vi "Get System Parameter by condition.vi"(8 "error in (no error)":errorcluster caption="错误输入（无错误）", 9 "Enable":bool[](array[boolean]), 10 "propertyName":string="BytesPersector", 11 "path":string="Win32_DiskDrive") -> (0 "error out":errorcluster caption="错误输出", 3 "Parameters":string[](array[string]))   [LabVIEW 2013, in "ManagementClass.lvclass"]
uses:
  ManagementClass.lvclass
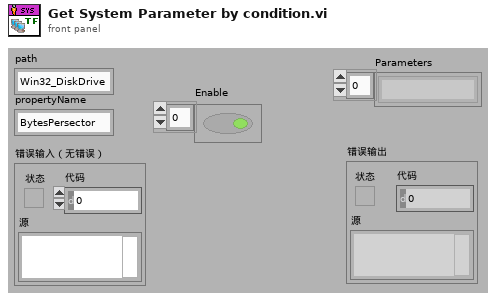
[diagram p1: front panel]
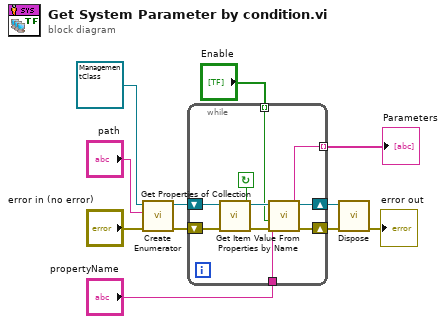
[diagram p0: block diagram]
diagram:
  n1 = call "Create Enumerator.vi"("error in (no error)"="error in (no error)", "path"="path", "ManagementClass 输入"=refnum<class "ManagementClass.lvclass"> refnum) -> ("error out"=w9:errorcluster, "ManagementClass 输出"=w10:refnum<class "ManagementClass.lvclass">)  [unwired: 7 in]
  n2 = while {
    shift-right: [w15] -> w7
    shift-left: w10 -> [w21]
    shift-right: [w16] -> w8
    shift-left: w9 -> [w18]
    tunnel: [w14] -> w2 mode=indexing
    tunnel: "propertyName" -> [w13]
    tunnel: "Enable" -> [w12] mode=indexing
    stop <- w20 continue-if-true
    n3 = call "Get Properties of Collection.vi"("error in (no error)"=w18, "ManagementClass 输入"=w21) -> ("error out"=w17:errorcluster, "非空"=w20:bool, "ManagementClass 输出"=w19:refnum<class "ManagementClass.lvclass">)  [unwired: 7 in]
    n4 = call "Get Item Value From Properties by Name.vi"("error in (no error)"=w17, "Enable"=w12, "PropertyName"=w13, "ManagementClass 输入"=w19) -> ("error out"=w16:errorcluster, "Value"=w14:string, "ManagementClass 输出"=w15:refnum<class "ManagementClass.lvclass">)  [unwired: 5 in]
  }
  "Parameters" <- w2
  n5 = call "Dispose.vi"("error in (no error)"=w8, "ManagementClass 输入"=w7) -> ("error out"=→"error out":errorcluster)  [unwired: 9 in]
